vi "GetVIData.vi"(8 "error in (no error)":errorcluster, 11 "VI in":refnum<vi>) -> (0 "error out":errorcluster, 1 "Get Conpane Image":T1, 2 "Array":string[](array[string]), 3 "VI out":refnum<vi>, 4 "Name":string, 5 "Panel":refnum<vi>)   [LabVIEW 2016, in "update vi properties.lvlib"]
uses:
  update vi properties.lvlib
  <vilib>/picture/picture.llb/imagedata.ctl
panel:
  # "Connector Pane"
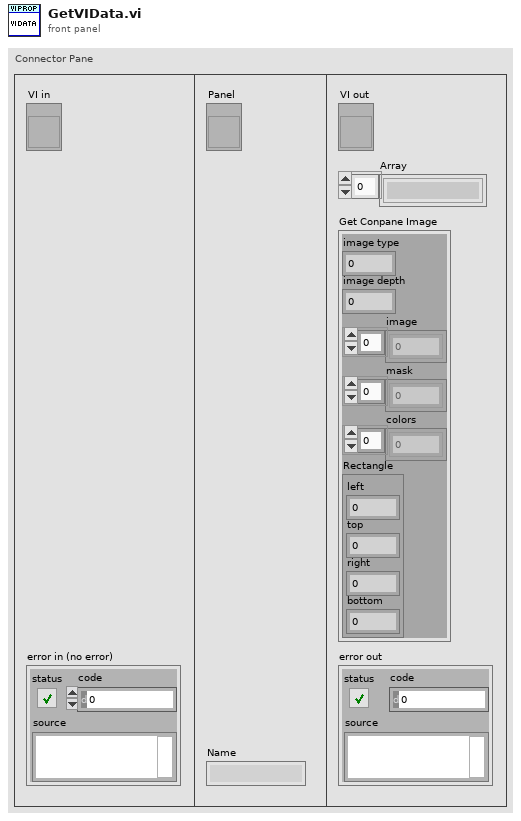
[diagram p1: front panel]
types:
  T1 = typedef "imagedata.ctl" = cluster{"image type":i32, "image depth":i32, "image":u8[], "mask":u8[], "colors":u32[], "Rectangle":cluster{"left":i16, "top":i16, "right":i16, "bottom":i16}}
  T2 = enum32{"invalid VI type", "Standard VI", "Control VI", "Global VI", "Polymorphic VI", "Configuration VI", "SubSystem", "Facade VI", "Method VI", "Statechart Diagram VI"}
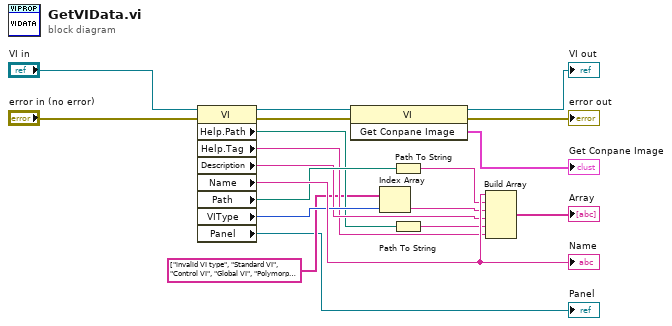
[diagram p0: block diagram]
diagram:
  n1 = property class="VI"(reference="VI in", error in="error in (no error)") -> (reference out=w3:refnum<vi>, error out=w4:errorcluster, "Help.Path"=w13:path, "Help.Tag"=w14:string, "Description"=w15:string, "Name"=w19:string, "Path"=w16:path, "VIType"=w17:T2, "Panel"=→"Panel":refnum<vi>)
  "Name" <- w19
  n2 = invoke class="VI" method="Get Conpane Image"(reference=w3, error in=w4) -> (reference out=→"VI out":refnum<vi>, error out=→"error out":errorcluster, "Get Conpane Image"=→"Get Conpane Image":T1)  [unwired: 1 in]
  n3 = Index Array(array=string[] ["invalid VI type", "Standard VI", "Control VI", "Global VI", "Polymorphic VI", "Configuration VI", "SubSystem", "Facade VI", "Method VI", "Statechart Diagram VI"] ("Strings []"), index=w17) -> (element=w10:string)
  n4 = Path To String(path=w16) -> (string=w11:string)
  n5 = Path To String(path=w13) -> (string=w9:string)
  n6 = Build Array(w19, w11, w10, w15, w9, w14) -> (→"Array":string[])
